vi "SetJSONData.vi"(0 "reference in":refnum<class "Progressbar.lvclass">, 1 "VI Reference":refnum<vi>, 2 "Value":string, 5 "error in (no error)":errorcluster) -> (14 "reference out":refnum<class "Progressbar.lvclass">, 19 "error out":errorcluster)   [LabVIEW 2014, in "FrontPanelPublisher.lvlib" / "Progressbar.lvclass"]
uses:
  Progressbar.lvclass
  Object_class/Object.lvclass
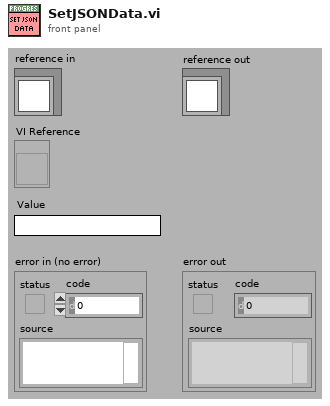
[diagram p1: front panel]
types:
  T1 = typedef "FrontPanelPublisher.lvlib/Object.lvclass/Attributes.ctl" = cluster{"UID":i32, "Type":string, "Coordinates":T2, "Reference":refnum<vi>}
  T2 = typedef "FrontPanelPublisher.lvlib/Object.lvclass/Coordinates.ctl" = cluster{"Left":i32, "Top":i32, "Height":u32, "Width":u32}
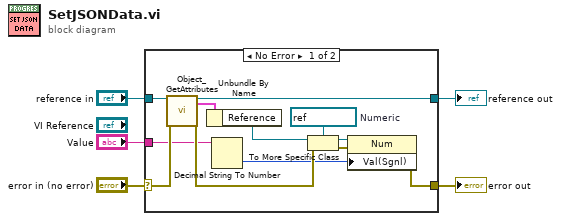
[diagram p0: block diagram]
diagram:
  n1 = case shown="No Error" "error in (no error)" {
    selector: "error in (no error)" -> [w17 w19]
    tunnel: [w16 w19] -> w4
    tunnel: [w11 w18] -> w2
    tunnel: "reference in" -> [w12 w18]
    tunnel: "Value" -> [w10 _]
    frame No Error {
      w6 = refnum<vi> refnum  # Numeric
      n2 = call "Object_GetAttributes.vi"("reference in"=w12, "error in (no error)"=w17) -> ("reference out"=w11:refnum<class "Progressbar.lvclass">, "Data"=w13:T1, "error out"=w15:errorcluster)  [unwired: 14 in, 1 out]
      n3 = Unbundle By Name(w13) -> ("Reference"=w9:refnum<vi>)
      n4 = Decimal String To Number(string=w10) -> (number=w8:i32)  [unwired: 2 in, 1 out]
      n5 = To More Specific Class(target class=w6, reference=w9, error in=w15) -> (specific class reference=w7:refnum<vi>, error out=w14:errorcluster)
      n6 = property class="Num"(reference=w7, error in=w14, "Val(Sgnl)"=w8) -> (error out=w16:errorcluster)  [unwired: 1 out]
    }
    frame Error {
    }
  }
  "error out" <- w4
  "reference out" <- w2
